vi "探头手动清洗.vi"(7 "校准参数":u16(ring) caption="校准参数：" items=["pH", "DO", "浊度", "电导率", "叶绿素a", "藻密度", "ORP", "DO2"], 8 "error in (no error)":errorcluster caption="错误输入（无错误）") -> (0 "error out":errorcluster caption="错误输出")   [LabVIEW 2016, in "斯坦道多参数.lvlib"]
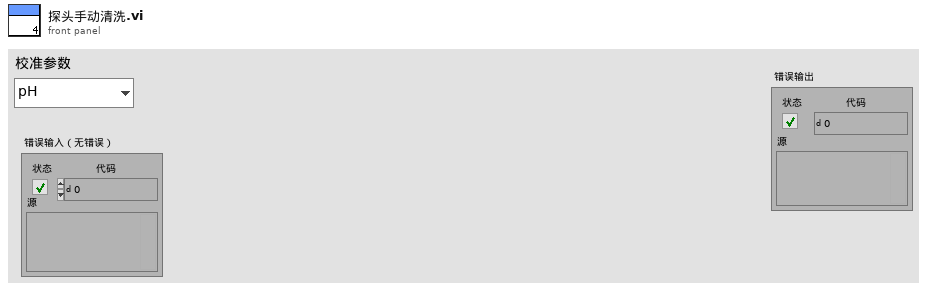
[diagram p1: front panel]
types:
  T1 = enum16{"NULL", "pH", "Cond", "DO", "Turb", "ORP"}
  T2 = enum16{"null", "pH", "DO", "浊度", "电导率", "叶绿素a", "藻密度"}
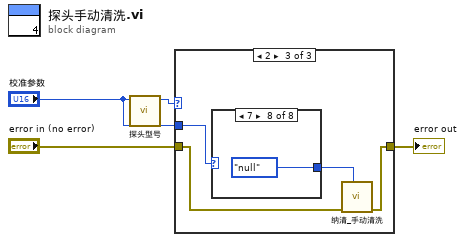
[diagram p0: block diagram]
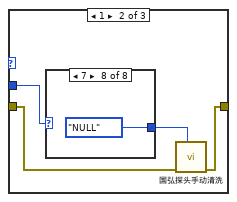
[diagram p3: hidden frame]
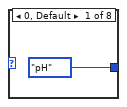
[diagram p4: hidden frame]
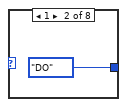
[diagram p5: hidden frame]
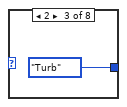
[diagram p6: hidden frame]
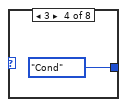
[diagram p7: hidden frame]
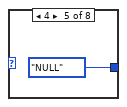
[diagram p8: hidden frame]
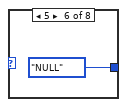
[diagram p9: hidden frame]
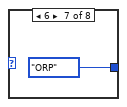
[diagram p10: hidden frame]
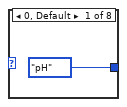
[diagram p11: hidden frame]
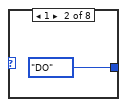
[diagram p12: hidden frame]
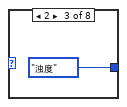
[diagram p13: hidden frame]
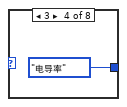
[diagram p14: hidden frame]
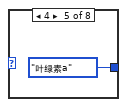
[diagram p15: hidden frame]
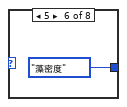
[diagram p16: hidden frame]
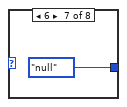
[diagram p17: hidden frame]
diagram:
  n1 = call "探头型号.vi"("校准参数"="校准参数") -> ("探头型号"=w4:u16)  [unwired: 8 in, 2 out]
  n2 = case shown="2" w4 {
    tunnel: "校准参数" -> [_ w9 w21]
    tunnel: "error in (no error)" -> [w5 w8 w19]
    tunnel: [w5 w6 w18] -> w1
    frame 0, Default {
    }
    frame 1 {
      n3 = case shown="7" w9 {
        tunnel: [T1."pH" ("探头") T1."DO" ("探头") T1."Turb" ("探头") T1."Cond" ("探头") T1."NULL" ("探头") T1."NULL" ("探头") T1."ORP" ("探头") T1."NULL" ("探头")] -> w7
        frame 0, Default {
        }
        frame 1 {
        }
        frame 2 {
        }
        frame 3 {
        }
        frame 4 {
        }
        frame 5 {
        }
        frame 6 {
        }
        frame 7 {
        }
      }
      n4 = call "国弘探头手动清洗.vi"("探头"=w7, "error in (no error)"=w8) -> ("error out"=w6:errorcluster)  [unwired: 8 in, 1 out]
    }
    frame 2 {
      n5 = case shown="7" w21 {
        tunnel: [T2."pH" ("探头") T2."DO" ("探头") T2."浊度" ("探头") T2."电导率" ("探头") T2."叶绿素a" ("探头") T2."藻密度" ("探头") T2."null" ("探头") T2."null" ("探头")] -> w20
        frame 0, Default {
        }
        frame 1 {
        }
        frame 2 {
        }
        frame 3 {
        }
        frame 4 {
        }
        frame 5 {
        }
        frame 6 {
        }
        frame 7 {
        }
      }
      n6 = call "纳清_手动清洗.vi"("探头"=w20, "error in (no error)"=w19) -> ("error out"=w18:errorcluster)  [unwired: 9 in]
    }
  }
  "error out" <- w1
